vi "Agua_llenado_sensor_00.vi"() -> ()   [LabVIEW 2022 SP3]
uses:
  <vilib>/Instr/_visa.llb/VISA Configure Serial Port (Instr).vi
panel:
  in  "Microcontrolador":string
  in  "ms/Ciclo":dbl=50.0
  out "mLs":dbl
  in  "Habilitado":bool
  out "Llenando...":bool
  out "Listo":bool=TRUE
  in  "500 ml":bool
  in  "300 ml":bool
  out "Vasito":dbl(slide) scale=0.0..500.0
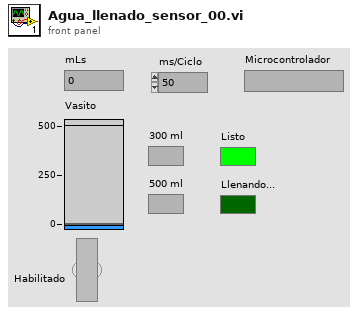
[diagram p1: front panel]
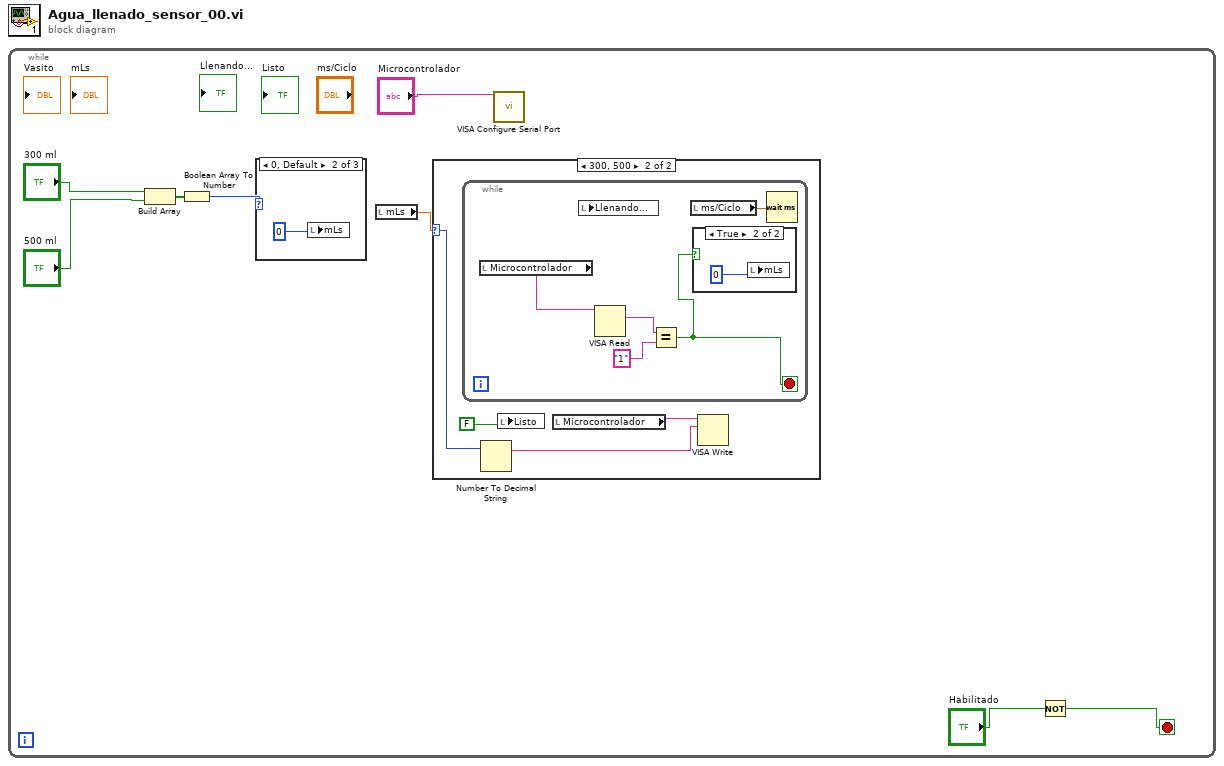
[diagram p0: block diagram]
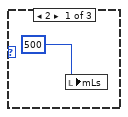
[diagram p2: hidden frame]
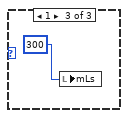
[diagram p3: hidden frame]
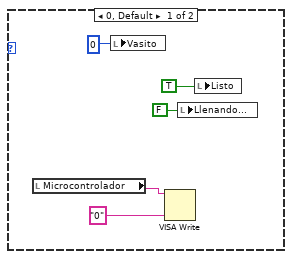
[diagram p4: hidden frame]
diagram:
  n1 = while {
    stop <- w3 stop-if-true
    n2 = Build Array("300 ml", "500 ml") -> (w8:bool[])
    n3 = Boolean Array To Number(Boolean array=w8) -> (number=w5:u32)
    n4 = case shown="0, Default" w5 {
      frame 2 {
        n5 = local write "mLs"(500) -> ()
      }
      frame 0, Default {
        n6 = local write "mLs"(0) -> ()
      }
      frame 1 {
        n7 = local write "mLs"(300) -> ()
      }
    }
    n8 = local read "mLs"() -> (w2:dbl)
    n9 = case shown="300, 500" w2 {
      selector: w2 -> [_ w18]
      frame 0, Default {
        n10 = local read "Microcontrolador"() -> (w13:string)
        n11 = local write "Vasito"(0) -> ()
        n12 = VISA Write(VISA resource name=w13, write buffer="0") -> ()  [unwired: 1 in, 3 out]
        n13 = local write "Llenando..."(FALSE) -> ()
        n14 = local write "Listo"(TRUE) -> ()
      }
      frame 300, 500 {
        n15 = while {
          stop <- w21 stop-if-true
          n16 = local read "Microcontrolador"() -> (w24:string)
          n17 = local read "Llenando..."() -> ()  [unwired: 1 in]
          n18 = VISA Read(VISA resource name=w24) -> (read buffer=w23:string)  [unwired: 2 in, 3 out]
          n19 = Equal?(x=w23, y="1") -> (x = y?=w21:bool)
          n20 = local read "ms/Ciclo"() -> (w25:dbl)
          n21 = case shown="True" w21 {
            frame False {
            }
            frame True {
              n22 = local write "mLs"(0) -> ()
            }
          }
          n23 = Wait (ms)(milliseconds to wait=w25) -> ()  [unwired: 1 out]
        }
        n24 = Number To Decimal String(number=w18) -> (decimal integer string=w17:string)  [unwired: 1 in]
        n25 = local write "Listo"(FALSE) -> ()
        n26 = local read "Microcontrolador"() -> (w19:string)
        n27 = VISA Write(VISA resource name=w19, write buffer=w17) -> ()  [unwired: 1 in, 3 out]
      }
    }
    n28 = call-poly "VISA Configure Serial Port"("VISA resource name"="Microcontrolador") -> ()  [unwired: 13 in, 2 out]
    n29 = Not(x="Habilitado") -> (.not. x?=w3:bool)
  }
